vi "TC_T_VtoC.vi"(11 "Thermocouple Voltage":dbl caption="热电偶电压" format="%0.6f") -> (3 "T(c)":dbl format="%#_16f")   [LabVIEW 2012]
doc: "功能：\n\nT型热电偶电压转换为摄氏度。\n\ncsxcs_366创建。"
uses:
  <vilib>/Analysis/polynomials.llb/Scalar Polynomial Evaluation (DBL).vi
  <vilib>/Analysis/NI_AALPro.lvlib
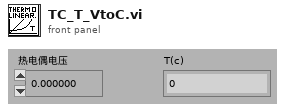
[diagram p1: front panel]
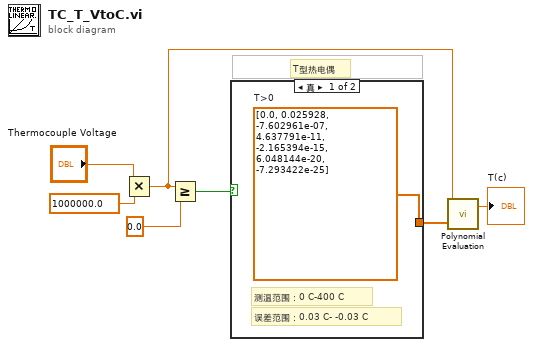
[diagram p0: block diagram]
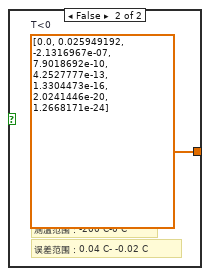
[diagram p2: hidden frame]
diagram:
  # "T型热电偶"
  n1 = Multiply(x="Thermocouple Voltage", y=1000000.0) -> (x*y=w3:dbl)
  n2 = Greater Or Equal?(x=w3, y=0.0) -> (x >= y?=w1:bool)
  n3 = case shown="真" w1 {
    tunnel: [w8 w9] -> w2
    frame True {
      w8 = dbl[] [0.0, 0.025928, -7.602961e-07, 4.637791e-11, -2.165394e-15, 6.048144e-20, -7.293422e-25]  # T>0
      # "误差范围：0.03 C- -0.03 C"
      # "测温范围：0 C-400 C"
    }
    frame False {
      w9 = dbl[] [0.0, 0.025949192, -2.1316967e-07, 7.9018692e-10, 4.2527777e-13, 1.3304473e-16, 2.0241446e-20, 1.2668171e-24]  # T<0
      # "误差范围：0.04 C- -0.02 C"
      # "测温范围：-200 C-0 C"
    }
  }
  n4 = call-poly <vilib>:"Polynomial Evaluation.vi"("P(x)"=w2, "a"=w3) -> ("P(a)"=→"T(c)":dbl)  [unwired: 1 out]
